vi "Q to Euler.vi"(6 "array":sgl[](array[numeric])) -> (0 "Roll":dbl, 1 "Yaw":dbl, 2 "Waveform Chart":cluster{"Yaw":dbl, "Pitch":dbl, "Roll":dbl}(graph), 3 "Pitch":dbl)   [LabVIEW 2015]
panel:
  # "This VI converts quanternion to Euler angles.\nnotice that the first three input variables (qx,qy,qz) represents the vector element,\nwhile the forth (qw) is the scalar element."
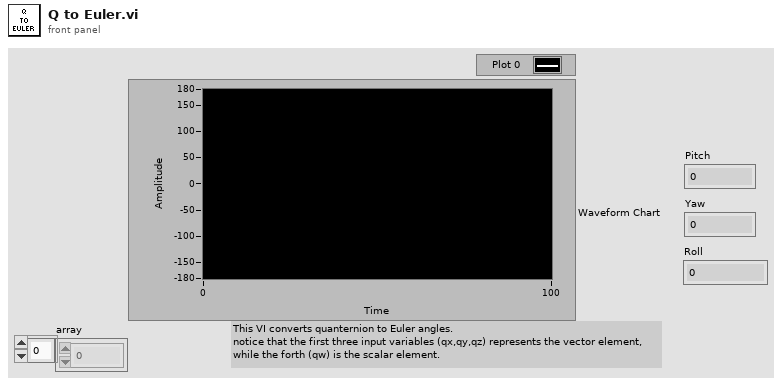
[diagram p1: front panel]
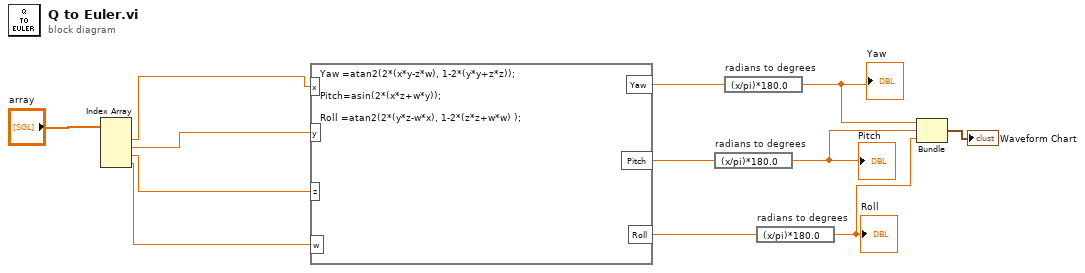
[diagram p0: block diagram]
diagram:
  n1 = Index Array(array="array") -> (element #1=w9:sgl, element #2=w8:sgl, element #3=w7:sgl, element #4=w6:sgl)  [unwired: 4 in]
  n2 = formula code="Yaw =atan2(2*(x*y-z*w),\t1-2*(y*y+z*z));\n\nPitch=asin(2*(x*z+w*y));\n\nRoll =atan2(2*(y*z-w*x), 1-2*(z*z+w*w) );"("x"=w9, "y"=w8, "z"=w7, "w"=w6) -> ("Yaw"=w12:dbl, "Pitch"=w11:dbl, "Roll"=w10:dbl)
  n3 = expression code="(x/pi)*180.0" "radians to degrees"(w11) -> (w4:dbl)
  "Pitch" <- w4
  n4 = expression code="(x/pi)*180.0" "radians to degrees"(w12) -> (w5:dbl)
  "Yaw" <- w5
  n5 = expression code="(x/pi)*180.0" "radians to degrees"(w10) -> (w3:dbl)
  "Roll" <- w3
  n6 = Bundle("Yaw"=w5, "Pitch"=w4, "Roll"=w3) -> (→"Waveform Chart":cluster{"Yaw":dbl, "Pitch":dbl, "Roll":dbl})  [unwired: 1 in]
